vi "SDCP TMC Encode and Decode test.vi"() -> ()   [LabVIEW 2020]
uses:
  Typedefs/SDCP TMC Param.ctl
panel:
  out "SDCP TMC out":T1
  out "Encoded frame":u8[](array[numeric])
  in  "SDCP TMC in":T1
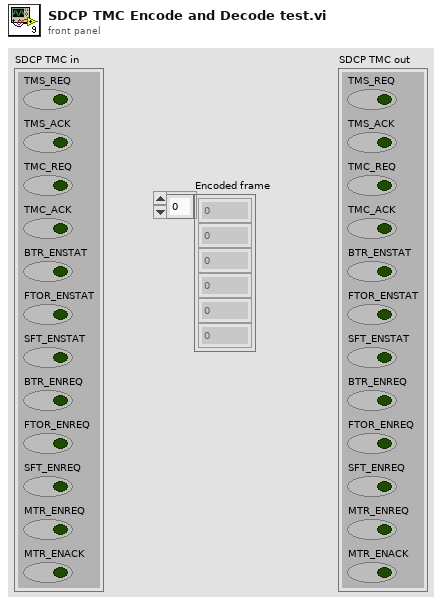
[diagram p1: front panel]
types:
  T1 = typedef "SDCP TMC Param.ctl" = cluster{"TMS_REQ":bool, "TMS_ACK":bool, "TMC_REQ":bool, "TMC_ACK":bool, "BTR_ENSTAT":bool, "FTOR_ENSTAT":bool, "SFT_ENSTAT":bool, "BTR_ENREQ":bool, "FTOR_ENREQ":bool, "SFT_ENREQ":bool, "MTR_ENREQ":bool, "MTR_ENACK":bool}
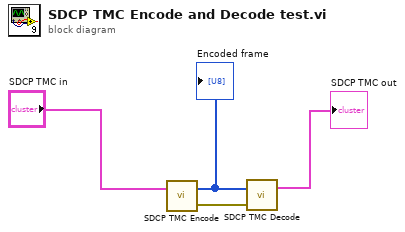
[diagram p0: block diagram]
diagram:
  n1 = call "SDCP TMC Encode.vi"("SDCP TMC Param"="SDCP TMC in") -> ("error out"=w3:errorcluster, "Encoded frame"=w2:u8[])  [unwired: 1 in]
  "Encoded frame" <- w2
  n2 = call "SDCP TMC Decode.vi"("error in (no error)"=w3, "Frame"=w2) -> ("SDCP TMC out"=→"SDCP TMC out":T1)  [unwired: 1 out]
